vi "ShooterPositioning-telop.vi"(8 "Encoder Val":dbl, 9 "Desired Distance":dbl, 10 "Touched the front?":bool, 11 "Start?":bool) -> (2 "Translational Set Val":dbl, 3 "Complete":bool)   [LabVIEW 2015]
uses:
  ShooterPositioningTelopStates.ctl
panel:
  out "Enum":T1
  in  "kd":dbl
  in  "Ki":dbl=0.14
  in  "Kp":dbl=0.00075
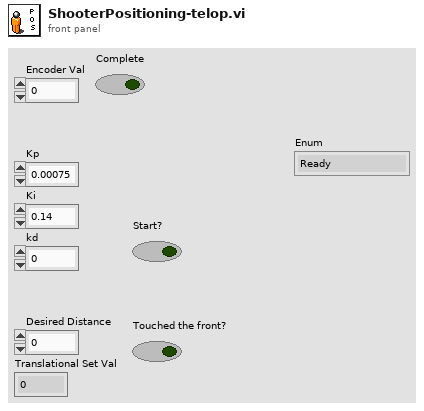
[diagram p1: front panel]
types:
  T1 = typedef "ShooterPositioningTelopStates.ctl" = enum16{"Ready", "To Castle", "Reset", "Back", "Shoot"}
  T2 = typedef "WPI_EncoderDevRef.ctl" = cluster{"DevStatus":errorcluster, "EncoderIndex":T3, "CounterIndex":T4, "DistancePerCount":dbl, "Decoding Type":T5}
  T3 = typedef "FPGA_EncoderIdx.ctl" = enum8{"Enc 0", "Enc 1", "Enc 2", "Enc 3", "Enc 4", "Enc 5", "Enc 6", "Enc 7", "Invalid"}
  T4 = typedef "FPGA_CounterCtrSystemIndex.ctl" = enum8{"Ctr 0", "Ctr 1", "Ctr 2", "Ctr 3", "Ctr 4", "Ctr 5", "Ctr 6", "Ctr 7", "Invalid"}
  T5 = typedef "WPI_EncoderType.ctl" = enum16{"1x", "2x", "4x"}
  T6 = typedef "WPI_GyroDevRef.ctl" = cluster{"DevStatus":errorcluster, "Analog Channel":T7, "Offset":dbl, "Gain (VoltsPerDegree/Second)":dbl, "Gyro Type":enum16{"Analog", "XRS450"}, "Handle":i32, "SPI Bus":T8, "Device Found":bool, "Sample Rate":dbl, "Calibrate On Open":bool}
  T7 = typedef "FPGA_AIChannel.ctl" = enum8{"AI 0", "AI 1", "AI 2", "AI 3", "AI MXP 0", "AI MXP 1", "AI MXP 2", "AI MXP 3", "Invalid"}
  T8 = typedef "spi_bus.ctl" = enum16{"SPI On-Board, CS0", "SPI On-Board, CS1", "SPI On-Board, CS2", "SPI On-Board, CS3", "SPI MXP", "Invalid"}
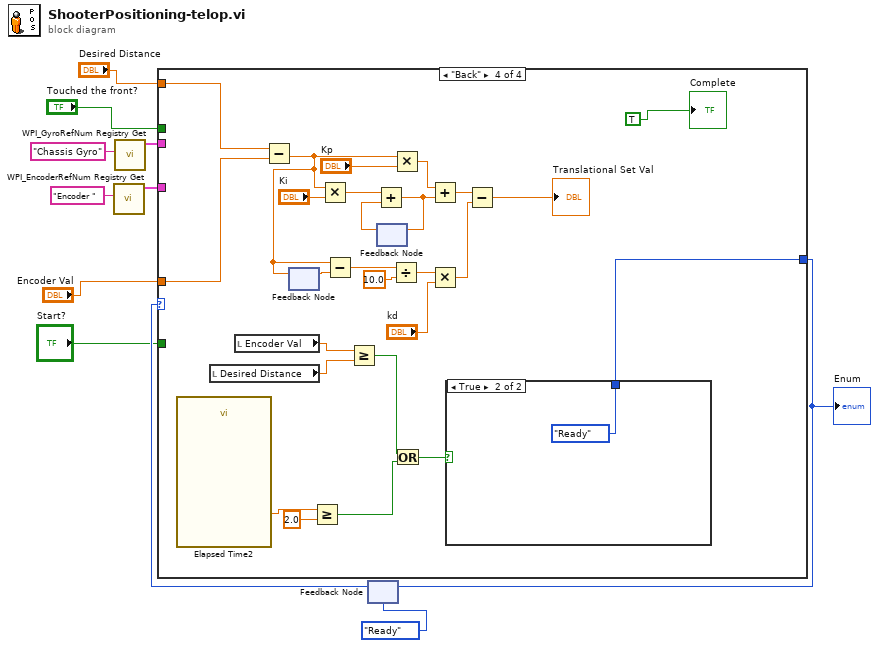
[diagram p0: block diagram]
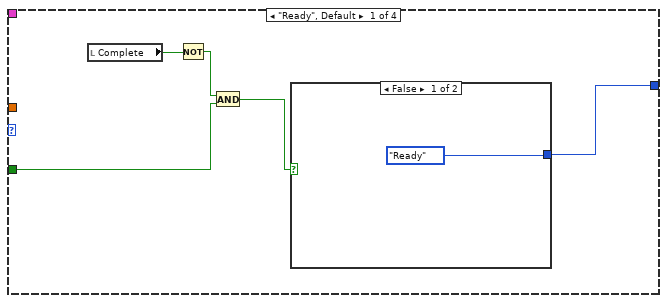
[diagram p2: hidden frame]
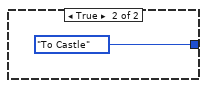
[diagram p3: hidden frame]
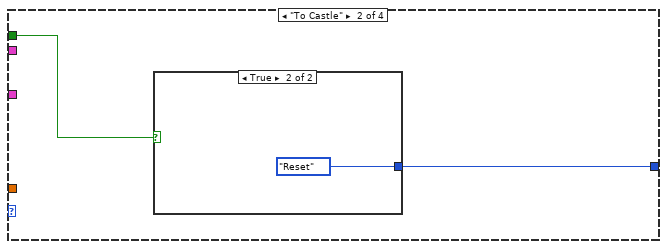
[diagram p4: hidden frame]
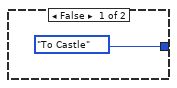
[diagram p5: hidden frame]
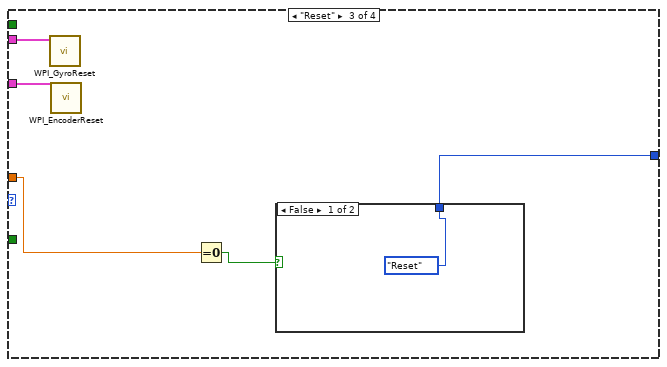
[diagram p6: hidden frame]
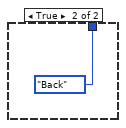
[diagram p7: hidden frame]
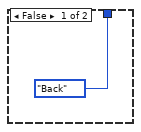
[diagram p8: hidden frame]
diagram:
  n1 = call <vilib>:"WPI_EncoderRefNum Registry Get.vi"("refnum name"="Encoder ") -> ("EncoderDevRef"=w1:T2)  [unwired: 9 in, 1 out]
  n2 = call <vilib>:"WPI_GyroRefNum Registry Get.vi"("refnum name"="Chassis Gyro") -> ("GyroDevRef"=w4:T6)  [unwired: 9 in, 1 out]
  n3 = feedback #1(ShooterPositioningTelopStates."Ready") -> (w10:T1)
  n4 = case shown="\"Back\"" w10 {
    tunnel: "Touched the front?" -> [_ w20 _ _]
    tunnel: [w16 w19 w25 w38] -> w8
    tunnel: "Start?" -> [w13 _ _ _]
    tunnel: "Desired Distance" -> [_ _ _ w37]
    tunnel: "Encoder Val" -> [_ _ w27 w36]
    tunnel: w4 -> [_ _ w24 _]
    tunnel: w1 -> [_ _ w23 _]
    frame "Ready", Default {
      n5 = local read "Complete"() -> (w15:bool)
      n6 = Not(x=w15) -> (.not. x?=w14:bool)
      n7 = And(x=w14, y=w13) -> (x .and. y?=w12:bool)
      n8 = case shown="False" w12 {
        tunnel: [ShooterPositioningTelopStates."Ready" ShooterPositioningTelopStates."To Castle"] -> w16
        frame False {
        }
        frame True {
        }
      }
    }
    frame "To Castle" {
      n9 = case shown="True" w20 {
        tunnel: [ShooterPositioningTelopStates."To Castle" ShooterPositioningTelopStates."Reset"] -> w19
        frame False {
        }
        frame True {
        }
      }
    }
    frame "Reset" {
      n10 = call <vilib>:"WPI_GyroReset.vi"("GyroDevRef"=w24) -> ()  [unwired: 9 in, 2 out]
      n11 = call <vilib>:"WPI_EncoderReset.vi"("EncoderDevRef"=w23) -> ()  [unwired: 9 in, 2 out]
      n12 = Equal To 0?(x=w27) -> (x = 0?=w26:bool)
      n13 = case shown="False" w26 {
        tunnel: [ShooterPositioningTelopStates."Reset" ShooterPositioningTelopStates."Back"] -> w25
        frame False {
        }
        frame True {
        }
      }
    }
    frame "Back" {
      n14 = call "Elapsed Time2"() -> ("Elapsed Time (s)"=w35:dbl)  [unwired: 12 in, 7 out]
      n15 = local read "Desired Distance"() -> (w39:dbl)
      n16 = local read "Encoder Val"() -> (w40:dbl)
      n17 = Subtract(x=w37, y=w36) -> (x-y=w41:dbl)
      n18 = feedback #2() -> (w53:dbl)  [unwired: 1 in]
      n19 = feedback-in #2(w41) -> ()
      n20 = Greater Or Equal?(x=w35, y=2.0) -> (x >= y?=w31:bool)
      n21 = Multiply(x=w41, y="Ki") -> (x*y=w55:dbl)
      n22 = Subtract(x=w41, y=w53) -> (x-y=w52:dbl)
      n23 = Greater Or Equal?(x=w40, y=w39) -> (x >= y?=w32:bool)
      n24 = feedback #3() -> (w54:dbl)  [unwired: 1 in]
      n25 = Add(x=w55, y=w54) -> (x+y=w48:dbl)
      n26 = feedback-in #3(w48) -> ()
      n27 = Divide(x=w52, y=10.0) -> (x/y=w50:dbl)
      n28 = Multiply(x=w41, y="Kp") -> (x*y=w49:dbl)
      n29 = Or(x=w32, y=w31) -> (x .or. y?=w33:bool)
      n30 = Add(x=w49, y=w48) -> (x+y=w47:dbl)
      n31 = Multiply(x=w50, y="kd") -> (x*y=w46:dbl)
      n32 = case shown="True" w33 {
        tunnel: [ShooterPositioningTelopStates."Back" ShooterPositioningTelopStates."Ready"] -> w38
        frame False {
        }
        frame True {
        }
      }
      n33 = Subtract(x=w47, y=w46) -> (x-y=→"Translational Set Val":dbl)
      "Complete" <- TRUE
    }
  }
  "Enum" <- w8
  n34 = feedback-in #1(w8) -> ()
